vi "CreateReadAccessor.vi"(6 "ClassPath":path, 7 "Write":bool, 8 "error in (no error)":errorcluster, 9 "properties":T1, 10 "PropDefFolder":refnum<vi>, 11 "LVClassLibrary Refnum":refnum<vi>) -> (0 "error out":errorcluster)   [LabVIEW 2013, in "GenLVOOP.lvclass"]
uses:
  GenLVOOP.lvclass
  baseClass/propertyDef.ctl
  baseClass/types.ctl
  baseClass/baseClass.lvclass
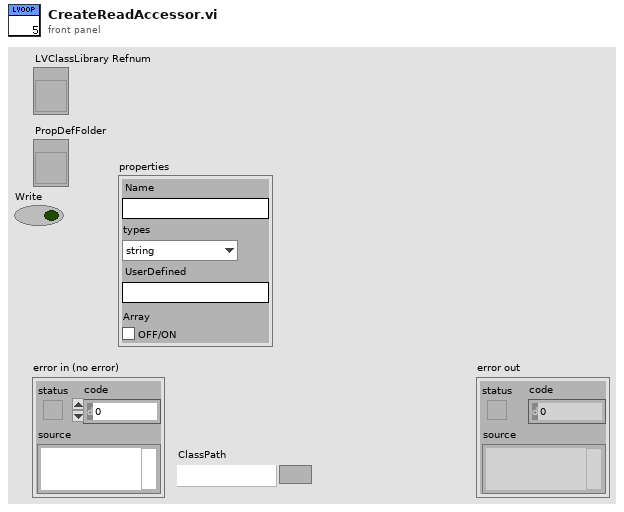
[diagram p1: front panel]
types:
  T1 = typedef "baseClass.lvclass/propertyDef.ctl" = cluster{"Name":string, "types":T2, "UserDefined":string, "Array":bool}
  T2 = typedef "baseClass.lvclass/types.ctl" = enum16{"string", "int", "decimal", "bool", "class", "enum"}
  T3 = enum32{"Invalid", "Standard", "Closed", "Hidden", "Minimized", "Maximized"}
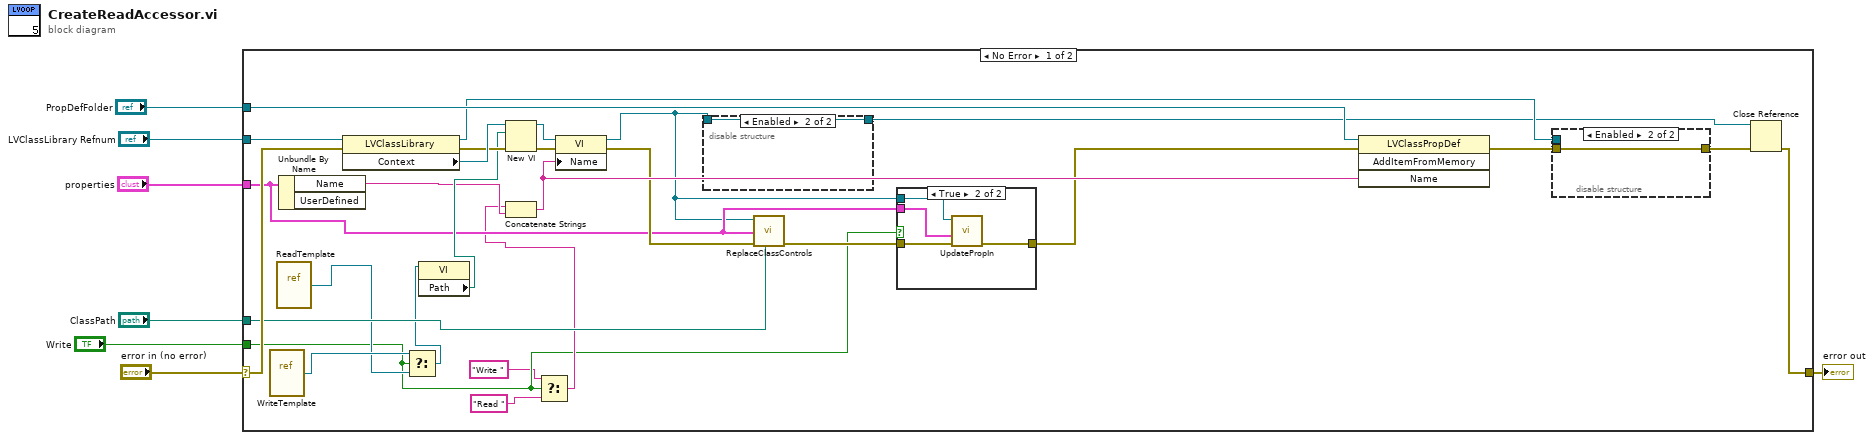
[diagram p0: block diagram]
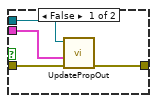
[diagram p2: hidden frame]
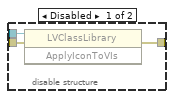
[diagram p3: hidden frame]
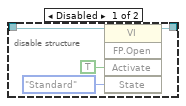
[diagram p4: hidden frame]
diagram:
  n1 = case shown="No Error" "error in (no error)" {
    selector: "error in (no error)" -> [w24 w53]
    tunnel: [w25 w53] -> w6
    tunnel: "LVClassLibrary Refnum" -> [w35 _]
    tunnel: "properties" -> [w18 _]
    tunnel: "PropDefFolder" -> [w30 _]
    tunnel: "ClassPath" -> [w20 _]
    tunnel: "Write" -> [w9 _]
    frame No Error {
      n2 = vi-ref "WriteTemplate.vi"() -> (w14:refnum<vi>)
      n3 = vi-ref "ReadTemplate.vi"() -> (w13:refnum<vi>)
      n4 = Unbundle By Name(w18) -> ("Name"=w19:string)  [unwired: 1 out]
      n5 = property class="LVClassLibrary"(reference=w35, error in=w24) -> (reference out=w27:refnum<vi>, error out=w33:errorcluster, "Context"=w34:refnum<vi>)
      n6 = Select(t=w14, s=w9, f=w13) -> (s? t:f=w12:refnum<vi>)
      n7 = property class="VI"(reference=w12) -> ("Path"=w23:path)  [unwired: 1 in, 2 out]
      n8 = New VI(8:w33, 10:w23, 11:w34) -> (0:w31:errorcluster, 3:w32:refnum<vi>)  [unwired: 4 in]
      n9 = Select(t="Write ", s=w9, f="Read ") -> (s? t:f=w10:string)
      n10 = Concatenate Strings(w10, w19) -> (w29:string)
      n11 = property class="VI"(reference=w32, error in=w31, "Name"=w29) -> (reference out=w17:refnum<vi>, error out=w21:errorcluster)
      n12 = disable-structure shown="Enabled" {
        disable-tunnel: w17 -> [w51 w52]
        disable-tunnel: [w48 w52] -> w22
        frame Disabled {
          n13 = invoke class="VI" method="FP.Open"(reference=w51, "Activate"=TRUE ("Activate?"), "State"=T3."Standard") -> (reference out=w48:refnum<vi>)  [unwired: 2 in, 4 out]
        }
        frame Enabled {
        }
      }
      n14 = call "ReplaceClassControls.vi"("ClassPath"=w20, "error in (no error)"=w21, "properties"=w18, "vi refnum"=w17) -> ("error out"=w16:errorcluster)  [unwired: 6 in, 1 out]
      n15 = case shown="True" w9 {
        tunnel: w18 -> [w39 w43]
        tunnel: w17 -> [w38 w42]
        tunnel: w16 -> [w37 w41]
        tunnel: [w36 w40] -> w15
        frame False {
          n16 = call "UpdatePropOut.vi"("error in (no error)"=w37, "properties"=w39, "vi refnum"=w38) -> ("error out"=w36:errorcluster)  [unwired: 8 in]
        }
        frame True {
          n17 = call "UpdatePropIn.vi"("error in (no error)"=w41, "properties"=w43, "vi refnum"=w42) -> ("error out"=w40:errorcluster)  [unwired: 8 in]
        }
      }
      n18 = invoke class="LVClassPropDef" method="AddItemFromMemory"(reference=w30, error in=w15, "Name"=w29) -> (error out=w28:errorcluster)  [unwired: 1 in, 3 out]
      n19 = disable-structure shown="Enabled" {
        disable-tunnel: w28 -> [w46 w47]
        disable-tunnel: w27 -> [w45 _]
        disable-tunnel: [w44 w47] -> w26
        frame Disabled {
          n20 = invoke class="LVClassLibrary" method="ApplyIconToVIs"(reference=w45, error in=w46) -> (error out=w44:errorcluster)  [unwired: 1 in, 2 out]
        }
        frame Enabled {
        }
      }
      n21 = Close Reference(reference=w22, error in (no error)=w26) -> (error out=w25:errorcluster)
    }
    frame Error {
    }
  }
  "error out" <- w6
